vi "Read Whole SEQ.vi"(0 "AOI List":u16[][](array[numeric]), 1 "# of Frames":i16, 2 "Output Sequence files handle":T1, 3 "error in":errorcluster, 4 "SEQ file refnum":refnum<file>, 5 "Header Info":T2, 7 "File name":string) -> (6 "# of frames read":i32, 8 "Frame height":i16, 9 "Frame width":i16, 10 "error out":errorcluster)   [LabVIEW 2016]
doc: "Supports 8-bit images only"
uses:
  Sequence files handle.ctt
  Seq file v 1/Offset table.ctl
  Seq file v 1/Offset.ctl
  Seq file v 1/file number.ctl
  GLIMPSE Globals.vi
panel:
  out "output variable":dbl
  in  "stop":bool
  out "Progress":i32(slide) scale=1.0..14.0
  # "Reading sequence file...."
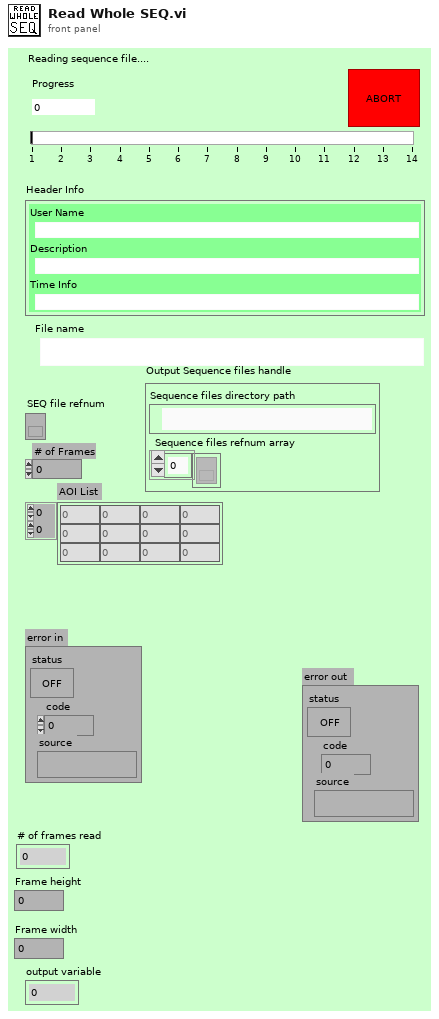
[diagram p1: front panel]
types:
  T1 = typedef "Sequence files handle.ctt" = cluster{"Sequence files directory path":path, "Sequence files refnum array":refnum<file>[]}
  T2 = cluster{"User Name":string, "Description":string, "Time Info":string}
  T3 = typedef "Offset table.ctl" = cluster{"offset":T4, "file number":T5}[]
  T4 = typedef "Offset.ctl" = i32
  T5 = typedef "file number.ctl" = u8
  T6 = typedef "IMAQ Image.ctl" = refnum<image>
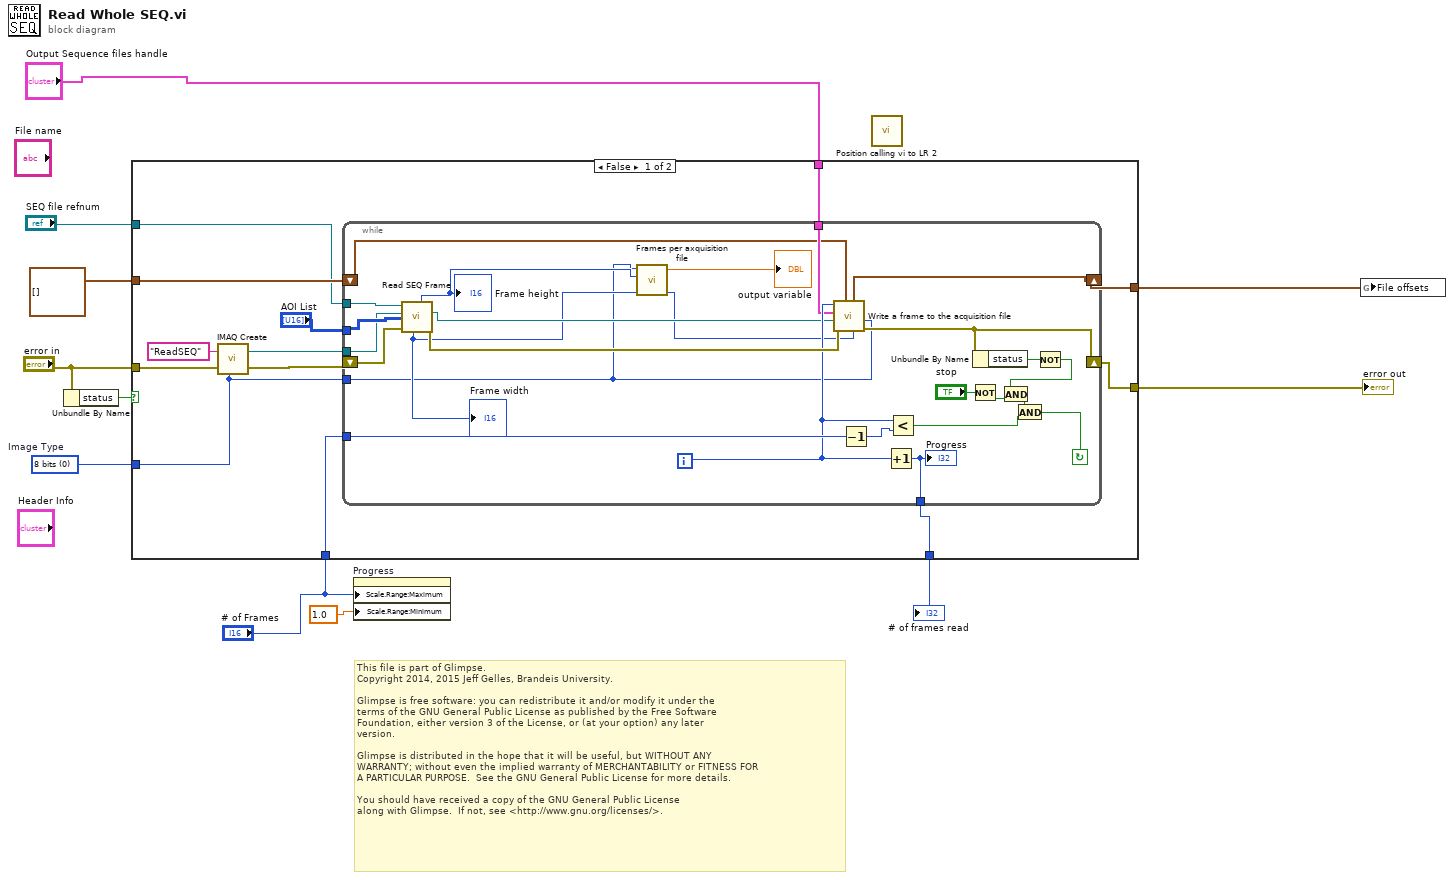
[diagram p0: block diagram]
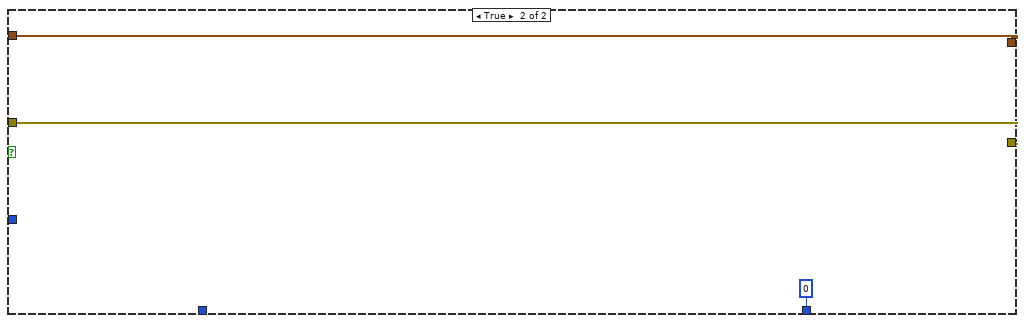
[diagram p2: hidden frame]
diagram:
  w3 = u32 0 items=["8 bits", "16 bits", "Float", "Complex", "RGB", "HSL"]  # Image Type
  # "This file is part of Glimpse. \nCopyright 2014, 2015 Jeff Gelles, Brandeis University.    \n\nGlimpse is free software: you can redistribute it and/or modify it under the \nterms of the GNU General Public License as published by the Free Software \nFoundation, either version 3 of the License, or (at your option) any later \nversion.\n\nGlimpse is distributed in the hope that it will be useful, but WITHOUT ANY \nWARRANTY; without even the implied warranty of MERCHANTABILITY or FITNESS FOR \nA PARTICULAR PURPOSE.  See the GNU General Public License for more details.\n\nYou should have received a copy of the GNU General Public License\nalong with Glimpse.  If not, see <http://www.gnu.org/licenses/>."
  n1 = Unbundle By Name("error in") -> ("status"=w6:bool)
  n2 = case shown="False" w6 {
    tunnel: "error in" -> [w18 w52]
    tunnel: "# of Frames" -> [w23 _]
    tunnel: [w22 w53] -> w9
    tunnel: [w19 w52] -> w8
    tunnel: T3 [] ("Offset table out") -> [w21 w53]
    tunnel: [w20 0] -> w4
    tunnel: w3 -> [w14 _]
    tunnel: "SEQ file refnum" -> [w13 _]
    tunnel: "Output Sequence files handle" -> [w12 _]
    frame False {
      n3 = call "IMAQ Create"("Image Name"="ReadSEQ", "Image Type"=w14, "error in (no error)"=w18) -> ("New Image"=w16:T6, "error out"=w17:errorcluster)  [unwired: 1 in, 1 out]
      n4 = while {
        tunnel: w23 -> [w48]
        shift-left: w17 -> [w49]
        shift-right: [w34] -> w19
        tunnel: "AOI List" -> [w50]
        tunnel: w12 -> [w39]
        shift-right: [w37] -> w22
        shift-left: w21 -> [w38]
        tunnel: w13 -> [w36]
        tunnel: [w35] -> w20
        tunnel: w16 -> [w30]
        tunnel: w14 -> [w25]
        i -> [w40]
        stop <- w45 continue-if-true
        n5 = call "Read SEQ Frame.vi"("error in (no error)"=w49, "AOI List"=w50, "Image Buffer In"=w30, "SEQ file refnum"=w36) -> ("error out"=w41:errorcluster, "Image Out"=w31:T6, "Output frame height"=w29:i16, "Output frame width"=w28:i16)  [unwired: 3 out]
        "Frame height" <- w29
        "Frame width" <- w28
        n6 = call "Frames per axquisition file.vi"("Output frame width"=w28, "Output frame height"=w29, "Pixel depth"=w25) -> ("Frames per acquisition file"=w27:i32, "Image size (pixels)"=→"output variable":dbl)  [unwired: 3 in]
        n7 = call "Write a frame to the acquisition file.vi"("Pixel depth"=w25, "Frames per acquisition file"=w27, "Offset table in"=w38, "error in"=w41, "Image In"=w31, "Sequence files handle"=w39, "Last frame number written in"=w40) -> ("error out"=w34:errorcluster, "Offset table out"=w37:T3)  [unwired: 3 out]
        n8 = Decrement(x=w48) -> (x-1=w32:i16)
        n9 = Increment(x=w40) -> (x+1=w35:i32)
        "Progress" <- w35
        n10 = Less?(x=w40, y=w32) -> (x < y?=w47:bool)
        n11 = Not(x="stop") -> (.not. x?=w43:bool)
        n12 = Unbundle By Name(w34) -> ("status"=w42:bool)
        n13 = Not(x=w42) -> (.not. x?=w33:bool)
        n14 = And(x=w33, y=w43) -> (x .and. y?=w44:bool)
        n15 = And(x=w44, y=w47) -> (x .and. y?=w45:bool)
      }
    }
    frame True {
    }
  }
  "error out" <- w8
  "# of frames read" <- w4
  n16 = property on="Progress" class="Slide (strict)"("Scale.Range:Maximum"="# of Frames", "Scale.Range:Minimum"=1.0 ("Minimum")) -> ()  [unwired: 2 in, 2 out]
  n17 = call "Position calling vi to LR 2.vi"() -> ()  [unwired: 2 in, 4 out]
  n18 = global write "GLIMPSE Globals.vi" "File offsets"(w9) -> ()
